vi "BIN_TO_DEC.vi"(10 "Before point?":bool, 11 "Array":dbl[](array[numeric])) -> (3 "output":dbl=2.0)   [LabVIEW 2023]
panel:
  out "size(s) 4":i32
  out "size(s) 2":i32
  out "Numeric 3":dbl=2.0
  out "size(s)":i32
  out "Numeric 2":dbl
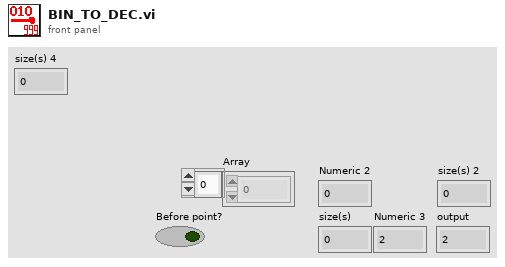
[diagram p1: front panel]
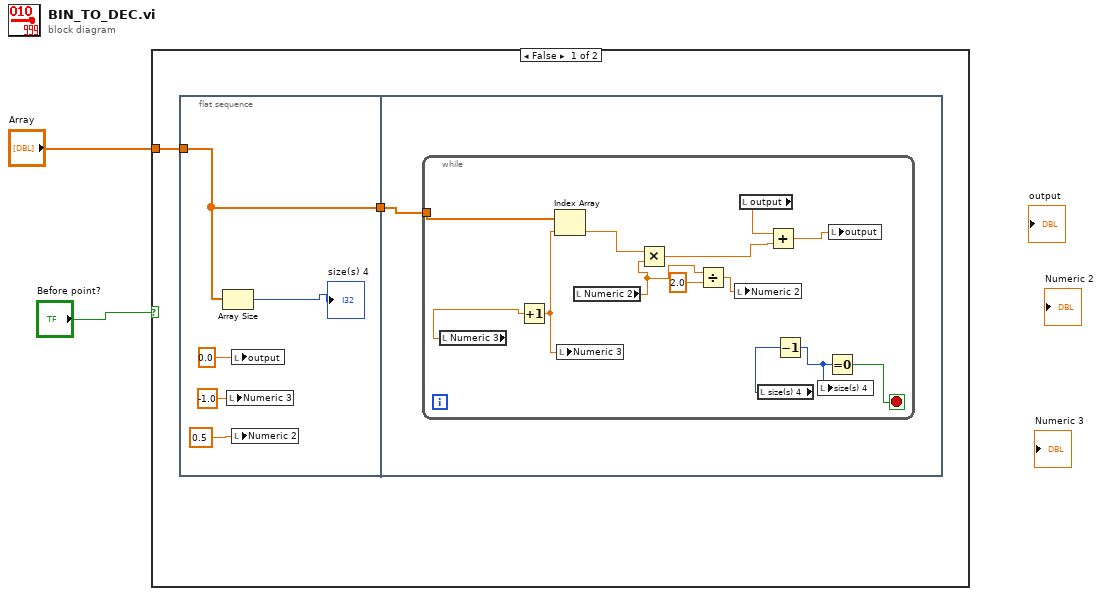
[diagram p0: block diagram]
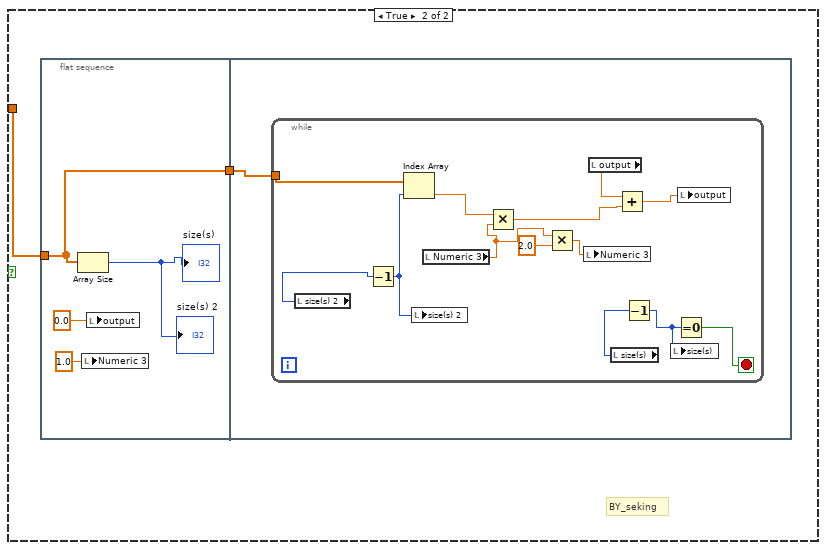
[diagram p2: hidden frame]
diagram:
  n1 = case shown="False" "Before point?" {
    tunnel: "Array" -> [w3 w24]
    frame False {
      n2 = flat-sequence {
        tunnel: [w6] -> w4
        tunnel: w3 -> [w6]
        tunnel: w4 -> [w10]
        frame #0 {
          n3 = Array Size(array=w6) -> (size(s)=→"size(s) 4":i32)
          n4 = local write "Numeric 3"(-1.0 ("Numeric 3")) -> ()
          n5 = local write "output"(0.0 ("Numeric 4")) -> ()
          n6 = local write "Numeric 2"(0.5 ("Numeric 2")) -> ()
        }
        frame #1 {
          n7 = while {
            tunnel: w10 -> [w23]
            stop <- w21 stop-if-true
            n8 = local read "Numeric 3"() -> (w18:dbl)
            n9 = Increment(x=w18) -> (x+1=w17:dbl)
            n10 = Index Array(array=w23, index=w17) -> (element=w19:dbl)
            n11 = local write "Numeric 3"(w17) -> ()
            n12 = local read "Numeric 2"() -> (w12:dbl)
            n13 = Multiply(x=w19, y=w12) -> (x*y=w11:dbl)
            n14 = Divide(x=w12, y=2.0) -> (x/y=w15:dbl)
            n15 = local write "Numeric 2"(w15) -> ()
            n16 = local read "output"() -> (w13:dbl)
            n17 = local read "size(s) 4"() -> (w22:i32)
            n18 = Add(x=w13, y=w11) -> (x+y=w14:dbl)
            n19 = Decrement(x=w22) -> (x-1=w20:i32)
            n20 = local write "size(s) 4"(w20) -> ()
            n21 = Equal To 0?(x=w20) -> (x = 0?=w21:bool)
            n22 = local write "output"(w14) -> ()
          }
        }
      }
    }
    frame True {
      # "BY_seking"
      n23 = flat-sequence {
        tunnel: w24 -> [w28]
        tunnel: [w28] -> w25
        tunnel: w25 -> [w30]
        frame #0 {
          n24 = Array Size(array=w28) -> (size(s)=→"size(s)" →"size(s) 2":i32)
          n25 = local write "Numeric 3"(1.0 ("Numeric 3")) -> ()
          n26 = local write "output"(0.0 ("Numeric 4")) -> ()
        }
        frame #1 {
          n27 = while {
            tunnel: w30 -> [w43]
            stop <- w41 stop-if-true
            n28 = local read "size(s) 2"() -> (w38:i32)
            n29 = Decrement(x=w38) -> (x-1=w37:i32)
            n30 = Index Array(array=w43, index=w37) -> (element=w39:dbl)
            n31 = local write "size(s) 2"(w37) -> ()
            n32 = local read "Numeric 3"() -> (w32:dbl)
            n33 = Multiply(x=w39, y=w32) -> (x*y=w31:dbl)
            n34 = Multiply(x=w32, y=2.0) -> (x*y=w35:dbl)
            n35 = local write "Numeric 3"(w35) -> ()
            n36 = local read "output"() -> (w33:dbl)
            n37 = local read "size(s)"() -> (w42:i32)
            n38 = Add(x=w33, y=w31) -> (x+y=w34:dbl)
            n39 = Decrement(x=w42) -> (x-1=w40:i32)
            n40 = local write "size(s)"(w40) -> ()
            n41 = Equal To 0?(x=w40) -> (x = 0?=w41:bool)
            n42 = local write "output"(w34) -> ()
          }
        }
      }
    }
  }
